vi "Group Arrays.vi"(9 "Grouping Size":dbl=3.0 format="%#_13g", 10 "length":i32, 11 "Averaged Values":dbl[][](array[numeric])) -> (2 "Array":dbl[](array[numeric]))   [LabVIEW 2018]
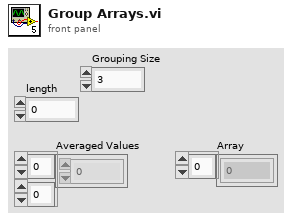
[diagram p1: front panel]
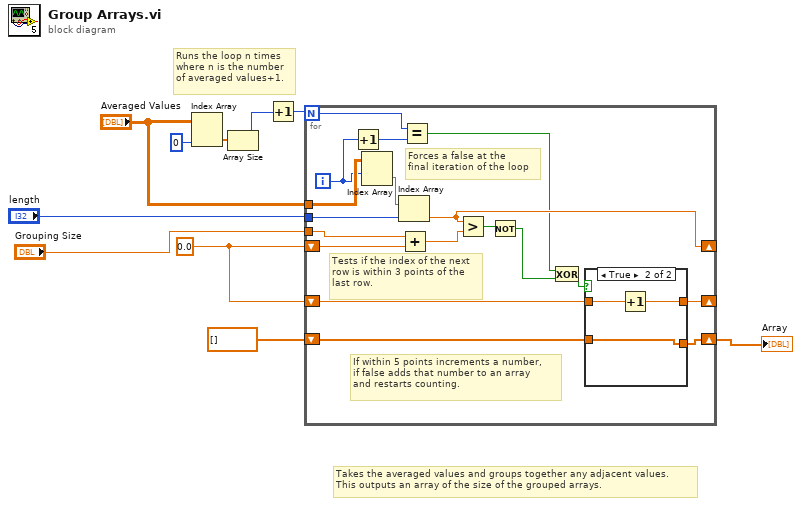
[diagram p0: block diagram]
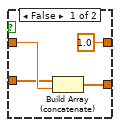
[diagram p2: hidden frame]
diagram:
  w3 = 0.0
  # "Runs the loop n times\nwhere n is the number\nof averaged values+1."
  # "Takes the averaged values and groups together any adjacent values. \nThis outputs an array of the size of the grouped arrays."
  n1 = Index Array(array="Averaged Values", index (col)=0 ("disabled index (col)")) -> (element=w4:dbl[])  [unwired: 1 in]
  n2 = Array Size(array=w4) -> (size(s)=w7:i32)
  n3 = Increment(x=w7) -> (x+1=w8:i32)
  n4 = for {
    N: w8 -> [w17]
    tunnel: "Averaged Values" -> [w22]
    tunnel: "length" -> [w23]
    shift-right: [w18] -> _
    shift-left: w3 -> [w19]
    shift-right: [w27] -> _
    shift-left: w3 -> [w26]
    shift-right: [w24] -> w9
    shift-left: dbl[] [] -> [w25]
    tunnel: "Grouping Size" -> [w11]
    i -> [w13]
    # "If within 5 points increments a number,\nif false adds that number to an array\nand restarts counting."
    # "Tests if the index of the next\nrow is within 3 points of the \nlast row."
    # "Forces a false at the \nfinal iteration of the loop"
    n5 = Increment(x=w13) -> (x+1=w12:i32)
    n6 = Index Array(array=w22, index (row)=w13) -> (element=w21:dbl[])  [unwired: 1 in]
    n7 = Index Array(array=w21, index=w23) -> (element=w18:dbl)
    n8 = Add(x=w11, y=w19) -> (x+y=w28:dbl)
    n9 = Equal?(x=w17, y=w12) -> (x = y?=w16:bool)
    n10 = Greater?(x=w18, y=w28) -> (0:w15:bool)
    n11 = Not(x=w15) -> (.not. x?=w14:bool)
    n12 = Exclusive Or(1:w14, 2:w16) -> (0:w20:bool)
    n13 = case shown="True" w20 {
      tunnel: w26 -> [w32 w35]
      tunnel: [1.0 w34] -> w27
      tunnel: w25 -> [w30 w33]
      tunnel: [w29 w33] -> w24
      frame False {
        n14 = Build Array (concatenate)(w30, w32) -> (w29:dbl[])
      }
      frame True {
        n15 = Increment(x=w35) -> (x+1=w34:dbl)
      }
    }
  }
  "Array" <- w9
